vi "NUC Calibration.vi"(0 "image in":refnum<class "MSC Image.lvclass">, 1 "image 2 in":refnum<class "MSC Image.lvclass">, 5 "error in (no error)":errorcluster) -> (14 "image out":refnum<class "MSC Image.lvclass">, 15 "image 2 out":refnum<class "MSC Image.lvclass">, 16 "NUC Table":T1, 19 "error out":errorcluster)   [LabVIEW 2016, in "MSC Image.lvclass"]
doc: "This Non-Uniformity Correction method is a twopoint calibration method. The input should be an image with maximum and minimum temperature. \n\nFor more information about this process please check the documentation."
uses:
  MSC Image.lvclass
  <vilib>/Analysis/NI_AALBase.lvlib
  <vilib>/Analysis/baseanly.llb/Mean (DBL).vi
  <vilib>/Analysis/NI_AALPro.lvlib
  controls/NUC Table.ctl
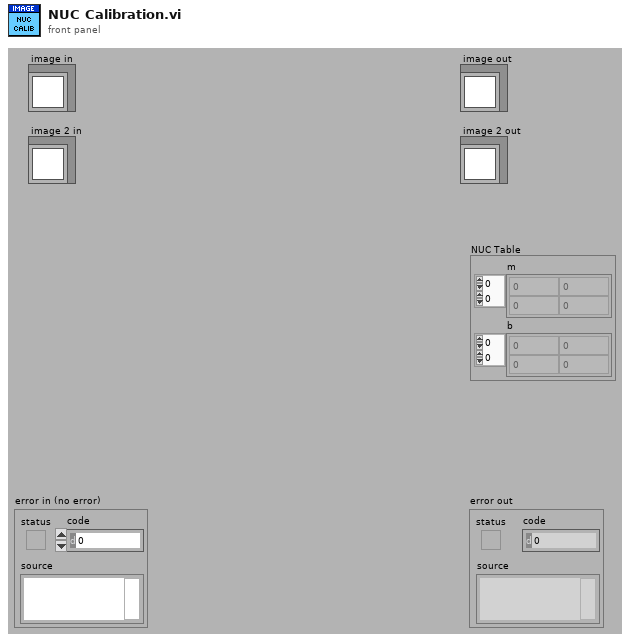
[diagram p1: front panel]
types:
  T1 = typedef "MSC Image.lvclass/NUC Table.ctl" = cluster{"m":dbl[][], "b":dbl[][]}
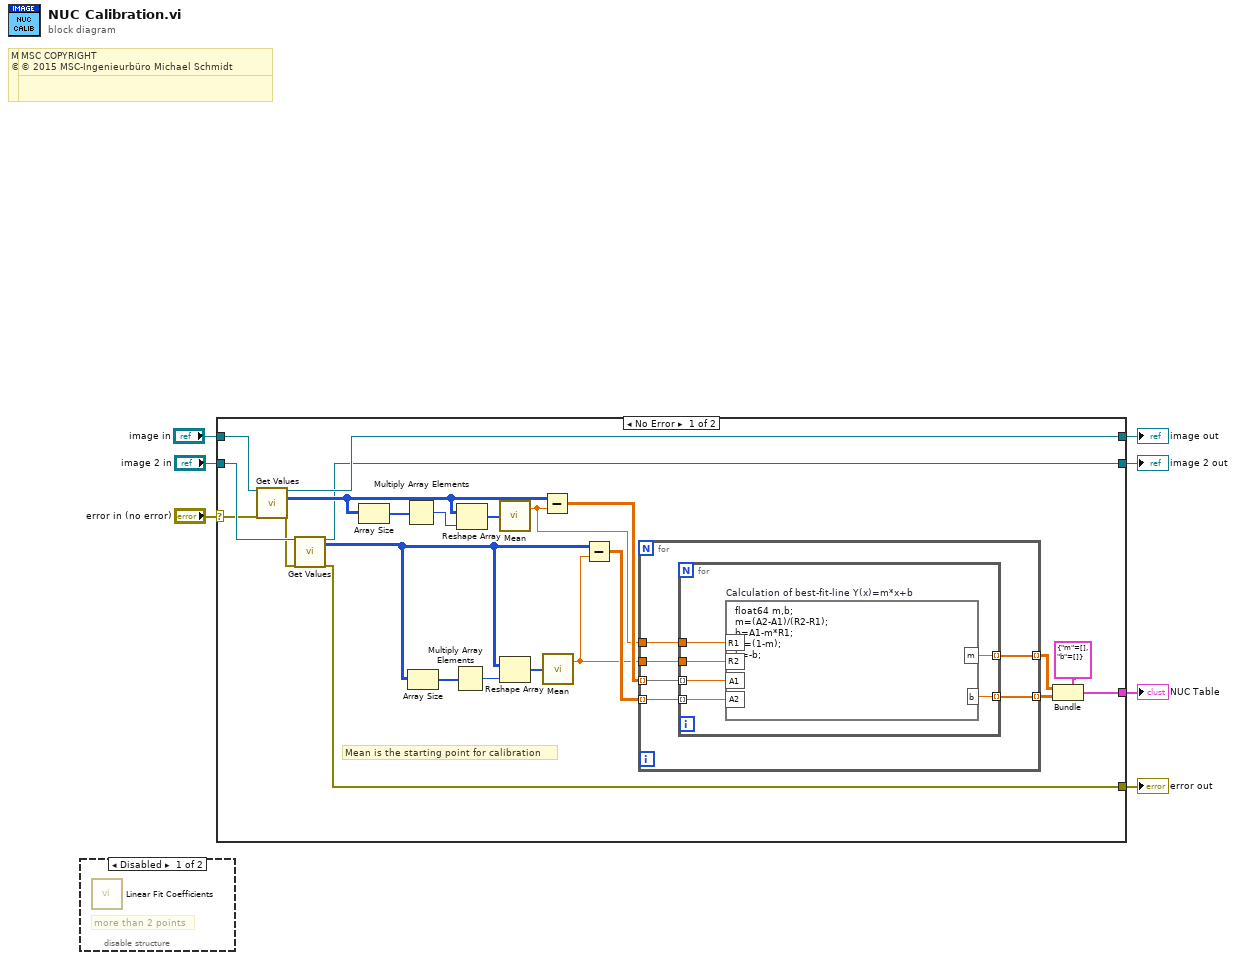
[diagram p0: block diagram]
diagram:
  # "MSC COPYRIGHT\n© 2016 MSC-Ingenieurbüro Michael Schmidt"
  # "MSC COPYRIGHT\n© 2016 MSC-Ingenieurbüro Michael Schmidt"
  # "MSC COPYRIGHT\n© 2015 MSC-Ingenieurbüro Michael Schmidt"
  # "MSC COPYRIGHT\n© 2015 MSC-Ingenieurbüro Michael Schmidt"
  n1 = disable-structure shown="Disabled" {
    frame Disabled {
      # "more than 2 points"
      n2 = call <vilib>:"Linear Fit Coefficients.vi"() -> ()  [unwired: 13 in, 3 out]
    }
    frame Enabled {
    }
  }
  n3 = case shown="No Error" "error in (no error)" {
    selector: "error in (no error)" -> [w10 w45]
    tunnel: [w9 w45] -> w2
    tunnel: [w14 w44] -> w4
    tunnel: "image in" -> [w15 w44]
    tunnel: "image 2 in" -> [w13 w43]
    tunnel: [w12 w43] -> w5
    tunnel: [w18 _] -> w1
    frame No Error {
      # "Mean is the starting point for calibration"
      n4 = call-dynamic "Get Values.vi"("image in"=w15, "error in (no error)"=w10) -> ("image out"=w14:refnum<class "MSC Image.lvclass">, "imageData U8"=w16:u8[][], "error out"=w11:errorcluster)  [unwired: 10 in, 5 out]
      n5 = call-dynamic "Get Values.vi"("image in"=w13, "error in (no error)"=w11) -> ("image out"=w12:refnum<class "MSC Image.lvclass">, "imageData U8"=w17:u8[][], "error out"=w9:errorcluster)  [unwired: 10 in, 5 out]
      n6 = Array Size(array=w16) -> (size(s)=w28:i32[])
      n7 = Multiply Array Elements(1:w28) -> (0:w29:i32)
      n8 = Array Size(array=w17) -> (size(s)=w26:i32[])
      n9 = Multiply Array Elements(1:w26) -> (0:w25:i32)
      n10 = Reshape Array(w16, w29) -> (w30:u8[])
      n11 = call-poly <vilib>:"Mean.vi"("X"=w30) -> ("mean"=w19:dbl)  [unwired: 1 out]
      n12 = Reshape Array(w17, w25) -> (w27:u8[])
      n13 = Subtract(x=w16, y=w19) -> (x-y=w21:dbl[][])
      n14 = call-poly <vilib>:"Mean.vi"("X"=w27) -> ("mean"=w20:dbl)  [unwired: 1 out]
      n15 = Subtract(x=w17, y=w20) -> (x-y=w22:dbl[][])
      n16 = for {
        tunnel: w20 -> [w36]
        tunnel: w19 -> [w35]
        tunnel: [w34] -> w24 mode=indexing
        tunnel: [w33] -> w23 mode=indexing
        tunnel: w21 -> [w32] mode=indexing
        tunnel: w22 -> [w31] mode=indexing
        n17 = for {
          tunnel: w36 -> [w42]
          tunnel: w35 -> [w41]
          tunnel: w32 -> [w37] mode=indexing
          tunnel: w31 -> [w38] mode=indexing
          tunnel: [w40] -> w33 mode=indexing
          tunnel: [w39] -> w34 mode=indexing
          n18 = formula code="float64 m,b;\nm=(A2-A1)/(R2-R1);\nb=A1-m*R1;\nm=(1-m);\nb=-b;" "Calculation of best-fit-line Y(x)=m*x+b"("R1"=w41, "R2"=w42, "A1"=w37, "A2"=w38) -> ("m"=w40:dbl, "b"=w39:dbl)
        }
      }
      n19 = Bundle(cluster=T1 {"m"=[], "b"=[]} ("NUC Table 2"), "m"=w23, "b"=w24) -> (w18:T1)
    }
    frame Error {
    }
  }
  "error out" <- w2
  "image out" <- w4
  "image 2 out" <- w5
  "NUC Table" <- w1
